vi "getMotorNames.vi"(11 "DeviceName":string) -> (3 "elements":string[](array[string]))   [LabVIEW 2013]
uses:
  Shared/MySQL/Preset Query Enum.ctl
  <userlib>/_OpenG.lib/array/array.llb/Filter 1D Array (String)__ogtk.vi
  <userlib>/_OpenG.lib/array/array.llb/Index 1D Array Elements (String)__ogtk.vi
  <userlib>/_OpenG.lib/array/array.llb/Remove Duplicates from 1D Array (String)__ogtk.vi
  <userlib>/_OpenG.lib/array/array.llb/Filter 1D Array with Scalar (String)__ogtk.vi
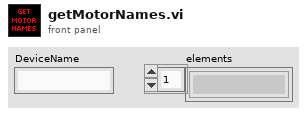
[diagram p1: front panel]
types:
  T1 = typedef "Preset Query Enum.ctl" = enum16{"Get Locations", "Get all IPs and MACs", "Get classes", "Get expt variables to set at scanstart for particular device", "Get expt devices and variables with start values", "Get expt devices and variables (with data to get)", "Get expt devices with data to get", "Get Expt devices and GUIs", "Get all devices basic properties", "Get Virtual Devices Core Info", "Get Expt names", "Get experiment basic properties", "Get experiment alarm variables", "Get MC Ports", "Get device network comm port", "Get devicetype lvclass path", "Get basic device properties", "Get Init Order", "Get all setable variables of a device", "Get device variable aliases", "Get force values of all settable variables", "Get all variables of a devicetype", "Get all variables of a device", "Get plotter details", "Get Saved Scans", "Get Scan Info", "GetGeneralGUIs", "Get expt for plotter", "Get plotter IDs from expt", "Get all devices", "Get all Virtual Devices", "Get all aliases", "Get variable and device info for Virtual Device", "GetItemLocatorIP", "Get IPs for GUIs", "Get DeviceType from Device", "GetLocalPortRange", "GetDevicePresetVariables", "Get Device Configuration", "GetAllPresetNames", "GetAllConfigurationNames", "GetPresetDeviceNames"}
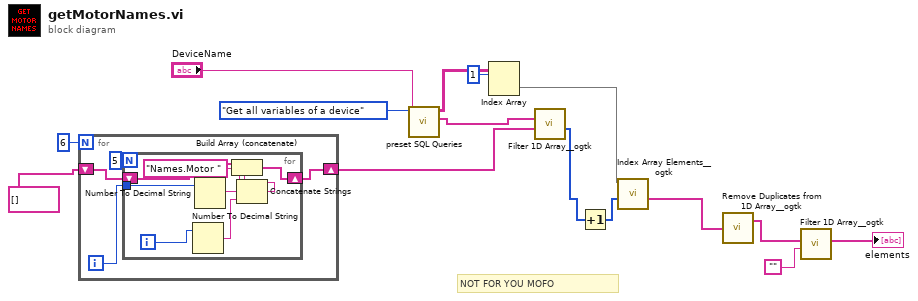
[diagram p0: block diagram]
diagram:
  # "NOT FOR YOU MOFO"
  n1 = for {
    N: 6 -> [_]
    shift-right: [w17] -> w10
    shift-left: string[] [] -> [w16]
    i -> [w18]
    n2 = for {
      N: 5 -> [_]
      tunnel: w18 -> [w27]
      shift-right: [w21] -> w17
      shift-left: w16 -> [w23]
      i -> [w26]
      n3 = Number To Decimal String(number=w26) -> (decimal integer string=w24:string)  [unwired: 1 in]
      n4 = Number To Decimal String(number=w27) -> (decimal integer string=w25:string)  [unwired: 1 in]
      n5 = Concatenate Strings("Names.Motor " ("string"), w25, w24) -> (w22:string)
      n6 = Build Array (concatenate)(w23, w22) -> (w21:string[])
    }
  }
  n7 = call "preset SQL Queries.vi"("Device/Devicetype name\n/Plotter.id/ScanName#"="DeviceName", "Preset Query"=Preset_Query_Enum."Get all variables of a device") -> ("1st column 1st data"=w7:string[], "data"=w11:string[][])  [unwired: 7 in, 1 out]
  n8 = Index Array(array=w11, index (col)=1 ("disabled index (col)")) -> (element=w13:string[])  [unwired: 1 in]
  n9 = call-poly <userlib>:"Filter 1D Array__ogtk.vi"("items to filter"=w10, "array"=w7) -> ("filtered item indices"=w14:i32[])  [unwired: 4 in, 1 out]
  n10 = Increment(x=w14) -> (x+1=w15:i32[])
  n11 = call-poly <userlib>:"Index Array Elements__ogtk.vi"("indices"=w15, "array"=w13) -> ("elements"=w4:string[])  [unwired: 9 in]
  n12 = call-poly <userlib>:"Remove Duplicates from 1D Array__ogtk.vi"("Input Array"=w4) -> ("Output Array"=w3:string[])  [unwired: 1 out]
  n13 = call-poly <userlib>:"Filter 1D Array__ogtk.vi"("items to filter"="", "array"=w3) -> ("filtered array"=→"elements":string[])  [unwired: 4 in, 1 out]
